vi "Calibrate.vi"(8 "error in":errorcluster, 11 "LTB-1 in":refnum<class "LTB-1.lvclass">) -> (0 "error out":errorcluster, 3 "LTB-1 out":refnum<class "LTB-1.lvclass">)   [LabVIEW 2018, in "LTB-1.lvlib" / "LTB-1.lvclass"]
doc: "This is a parent VI. The children VI will overwrite this with the correct calls for calibration.\n\nAuthor: Ron Dexter\nCompany: Luminar\nModified: 5/20/2018"
uses:
  LTB-1.lvclass
  C:/AME Test Engineering/LabVIEW/PPLs/EXFO/Parent/EXFO.lvlibp/EXFO.lvclass
  LTB-1.lvclass/LTB-1.ctl
  PPLs/EXFO/Parent/EXFO.lvlibp/Methods/Read Resource.vi
  3150 Driver/3150.lvlib
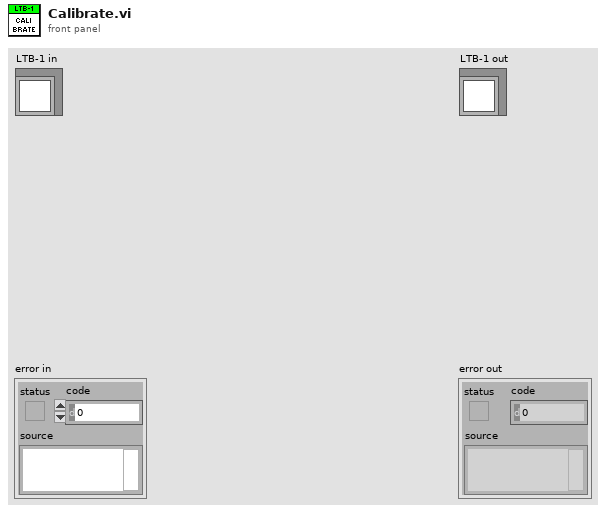
[diagram p1: front panel]
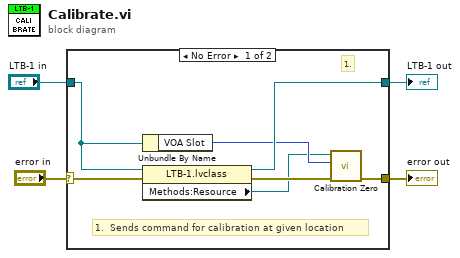
[diagram p0: block diagram]
diagram:
  n1 = case shown="No Error" "error in" {
    selector: "error in" -> [w10 w13]
    tunnel: "LTB-1 in" -> [w9 w12]
    tunnel: [w11 w12] -> w3
    tunnel: [w7 w13] -> w2
    frame No Error {
      # "1.  Sends command for calibration at given location"
      # "1."
      n2 = Unbundle By Name(w9) -> ("VOA Slot"=w6:i16)
      n3 = property class="LTB-1.lvclass"(reference=w9, error in=w10) -> (reference out=w11:refnum<class "LTB-1.lvclass">, error out=w8:errorcluster, "Methods:Resource"=w5:refnum<visa-resource-name>)
      n4 = call "Calibration Zero.vi"("error in (no error)"=w8, "Platform Slot Number (10)"=w6, "VISA resource name"=w5) -> ("error out"=w7:errorcluster)  [unwired: 7 in, 1 out]
    }
    frame Error {
    }
  }
  "error out" <- w2
  "LTB-1 out" <- w3
